vi "X-Y Go.vi"() -> ()   [LabVIEW 2010]
panel:
  out "y-axis":bool
  out "x-axis":bool
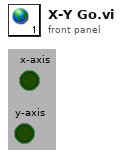
[diagram p1: front panel]
diagram:
